vi "Air Thermal Conductivity.vi"(11 "Temperature (C)":dbl) -> (3 "Thermal Conductivity (W/m-K)":dbl)   [LabVIEW 2019]
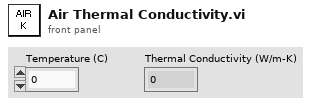
[diagram p1: front panel]
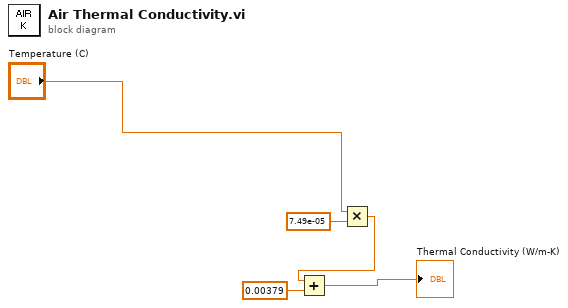
[diagram p0: block diagram]
diagram:
  n1 = Multiply(x="Temperature (C)", y=7.49e-05) -> (x*y=w3:dbl)
  n2 = Add(x=w3, y=0.00379) -> (x+y=→"Thermal Conductivity (W/m-K)":dbl)
